vi "Parse Channels.vi"(4 "tx channel handle array":u32[](array[numeric]), 5 "ScheduledSDI":bool, 6 "rx channel handle array":u32[](array[numeric]), 7 "FIFO Idx Qs":T1, 8 "error in (no error)":errorcluster, 9 "Access":T3, 10 "Section GUID":string, 11 "Device Reference in":T2 format="%.0x") -> (0 "error out":errorcluster, 1 "Section BaseRate":i32, 2 "Section Data":T4[](array[typedef]) {"Labels Settings"."Label" format="%.0o"}, 3 "Device Reference out":T2 format="%.0x")   [LabVIEW 2011, in "AIT 429 Custom Device.lvlib"]
uses:
  AIT 429 Custom Device.lvlib
  RT Controls/RT HW Channel.ctl
  RT Controls/RT Label Settings.ctl
  Controls and Global/Label.ctl
  Controls and Global/transferPeriod.ctl
  RT Controls/Driver Data.ctl
  RT Controls/RT Word Settings.ctl
  <vilib>/NI Veristand/Custom Device API/Block Data Reference.ctl
  <vilib>/NI Veristand/Custom Device API/Data Reference.ctl
  RT Controls/RT Param Setting.ctl
  Controls and Global/Start Bit.ctl
  Controls and Global/Number of Bits.ctl
  Controls and Global/TransferType.ctl
  <vilib>/NI Veristand/Custom Device API/Data Access Type.ctl
  <vilib>/NI Veristand/Custom Device API/Custom Device Item Ref.ctl
  RT Controls/FIFO Idx Qs.ctl
  <vilib>/NI Veristand/Custom Device Tools/Custom Device Utility Library/NI VeriStand - Search for Item by GUID.vi
  Controls and Global/Global.vi
  <vilib>/NI Veristand/Custom Device API/Get Item Property (U16).vi
  <vilib>/NI Veristand/Custom Device API/Get Item Property (U32).vi
  <instrlib>/AIT 429/Public/Tx/Data/AIT 429 Set Scheduled Label Transfer Period.vi
  <vilib>/NI Veristand/Custom Device API/Get Item Property (Double).vi
  <vilib>/NI Veristand/Custom Device Tools/Custom Device Utility Library/Custom Device Utility Library.lvlib
  <vilib>/NI Veristand/Custom Device API/Custom Device API.lvlib
  <userlib>/ARINC-429/Owl429.lvlib
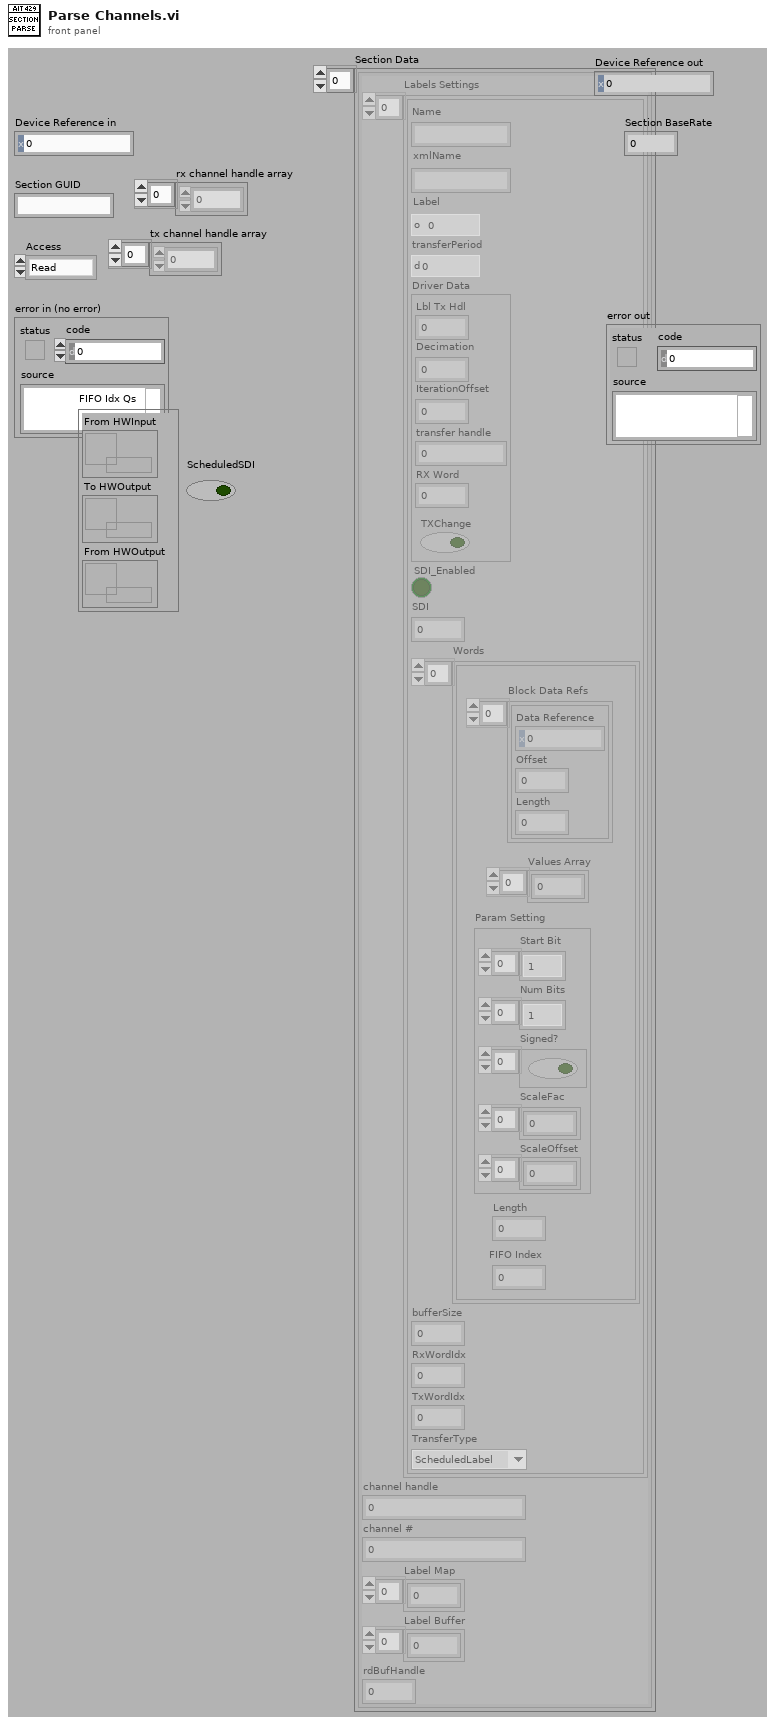
[diagram p1: front panel]
types:
  T1 = typedef "AIT 429 Custom Device.lvlib/FIFO Idx Qs.ctl" = cluster{"From HWInput":refnum<queue>, "To HWOutput":refnum<queue>, "From HWOutput":refnum<queue>}
  T2 = typedef "Custom Device API.lvlib/Custom Device Item Ref.ctl" = u64
  T3 = typedef "Custom Device API.lvlib/Data Access Type.ctl" = enum16{"Read", "Write"}
  T4 = typedef "AIT 429 Custom Device.lvlib/RT HW Channel.ctl" = cluster{"Labels Settings":T5[], "channel handle":u32, "channel #":u16, "Label Map":i32[], "Label Buffer":u32[], "rdBufHandle":u32}
  T5 = typedef "AIT 429 Custom Device.lvlib/RT Label Settings.ctl" = cluster{"Name":string, "xmlName":string, "Label":T6, "transferPeriod":T7, "Driver Data":T8, "SDI_Enabled":bool, "SDI":u8, "Words":T9[], "bufferSize":u32, "RxWordIdx":i32, "TxWordIdx":i32, "TransferType":T15}
  T6 = typedef "AIT 429 Custom Device.lvlib/Label.ctl" = u8
  T7 = typedef "AIT 429 Custom Device.lvlib/transferPeriod.ctl" = u32
  T8 = typedef "AIT 429 Custom Device.lvlib/Driver Data.ctl" = cluster{"Lbl Tx Hdl":u32, "Decimation":i32, "IterationOffset":i32, "transfer handle":u32, "RX Word":u32, "TXChange":bool}
  T9 = typedef "AIT 429 Custom Device.lvlib/RT Word Settings.ctl" = cluster{"Block Data Refs":T10[], "Values Array":dbl[], "Length":i32, "FIFO Index":i32, "Param Setting":T12}
  T10 = typedef "Custom Device API.lvlib/Block Data Reference.ctl" = cluster{"Data Reference":T11, "Offset":i32, "Length":i32}
  T11 = typedef "Custom Device API.lvlib/Data Reference.ctl" = i32
  T12 = typedef "AIT 429 Custom Device.lvlib/Rt Param Setting.ctl" = cluster{"Start Bit":T13[], "Num Bits":T14[], "Signed?":bool[], "ScaleFac":dbl[], "ScaleOffset":dbl[]}
  T13 = typedef "AIT 429 Custom Device.lvlib/Start Bit.ctl" = i32
  T14 = typedef "AIT 429 Custom Device.lvlib/Number of Bits.ctl" = i32
  T15 = typedef "AIT 429 Custom Device.lvlib/TransferType.ctl" = enum16{"ScheduledLabel", "Acyclic", "Block", "Strobe"}
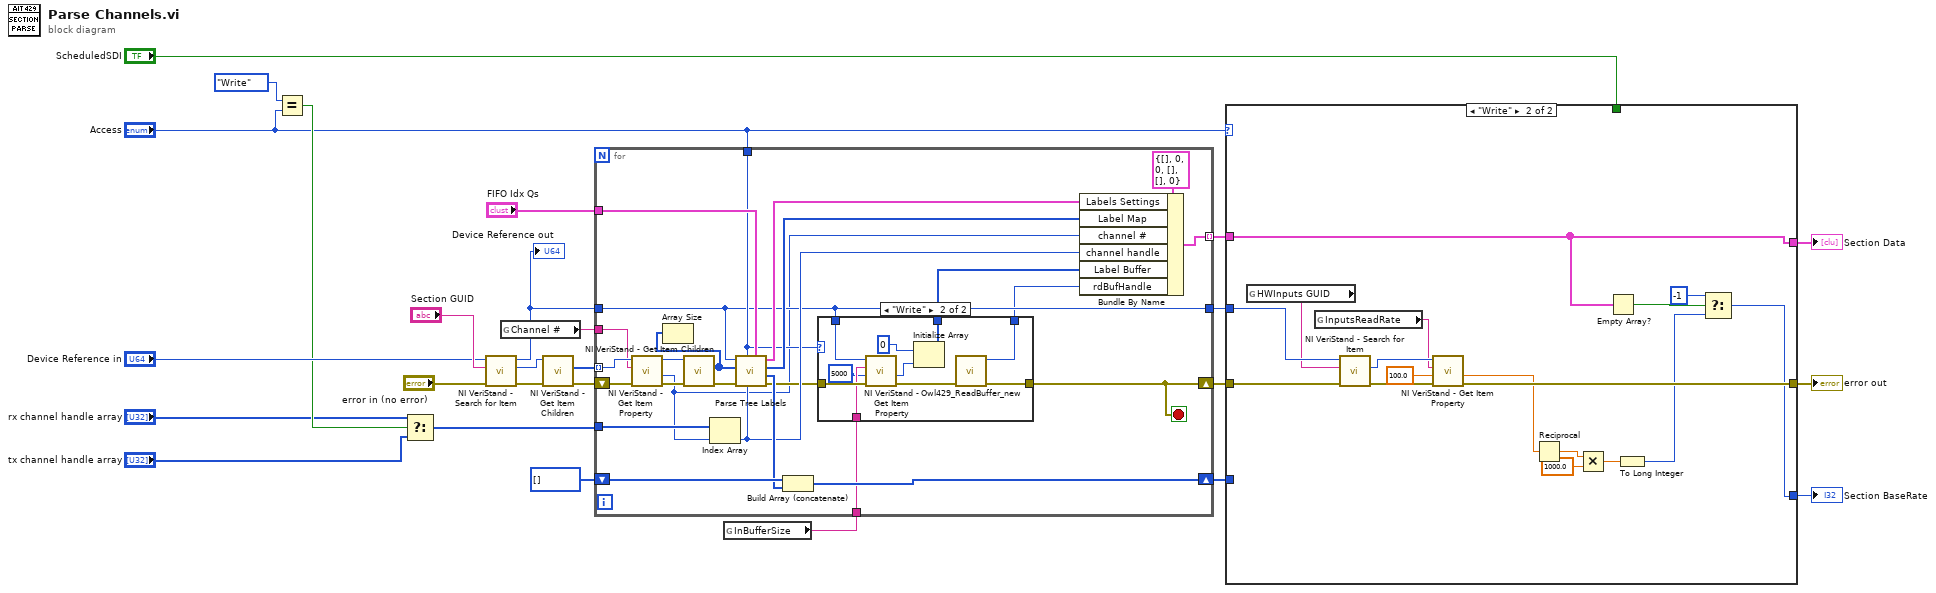
[diagram p0: block diagram]
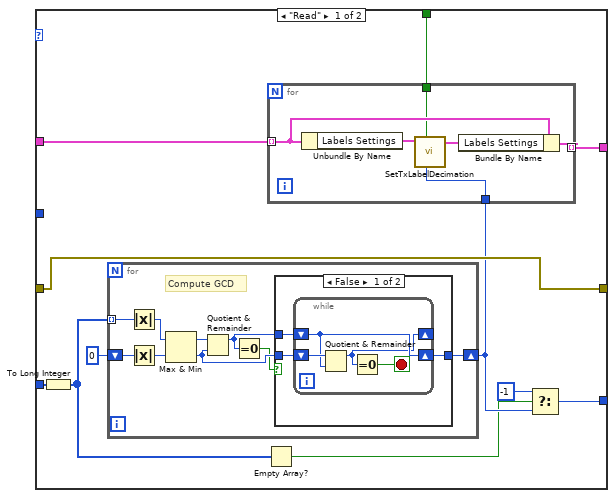
[diagram p2: hidden frame]
diagram:
  n1 = Equal?(x=Data_Access_Type."Write" ("y"), y="Access") -> (x = y?=w11:bool)
  n2 = Select(t="rx channel handle array", s=w11, f="tx channel handle array") -> (s? t:f=w8:u32[])
  n3 = call-poly <vilib>:"NI VeriStand - Search for Item.vi"("error in"="error in (no error)", "Item GUID"="Section GUID", "Section Ref in"="Device Reference in") -> ("error out"=w21:errorcluster, "Item Ref"=w22:T2, "Section Ref out"=w26:T2)  [unwired: 5 in, 1 out]
  "Device Reference out" <- w26
  n4 = global read "Global.vi" "Channel #"() -> (w3:string)
  n5 = call <vilib>:"NI VeriStand - Get Item Children.vi"("error in (no error)"=w21, "Item Ref in"=w22) -> ("error out"=w25:errorcluster, "Child Refs"=w24:T2[])  [unwired: 6 in, 2 out]
  n6 = global read "Global.vi" "InBufferSize"() -> (w2:string)
  n7 = for {
    tunnel: w24 -> [w42] mode=indexing
    tunnel: "Access" -> [w36]
    tunnel: w26 -> [w34]
    tunnel: [w49] -> w16 mode=indexing
    shift-right: [w30] -> w6
    shift-left: w25 -> [w44]
    shift-right: [w45] -> w17
    shift-left: u32[] [] -> [w47]
    tunnel: w8 -> [w39]
    tunnel: "FIFO Idx Qs" -> [w40]
    tunnel: [w34] -> w4
    tunnel: w3 -> [w33]
    tunnel: w2 -> [w32]
    stop <- w30 stop-if-true
    n8 = call-poly <vilib>:"NI VeriStand - Get Item Property.vi"("error in (no error)"=w44, "Property Name"=w33, "Item Ref in"=w42) -> ("error out"=w43:errorcluster, "Value"=w28:u16, "Item Ref out"=w41:T2)  [unwired: 5 in, 1 out]
    n9 = call <vilib>:"NI VeriStand - Get Item Children.vi"("error in (no error)"=w43, "Item Ref in"=w41) -> ("error out"=w48:errorcluster, "Child Refs"=w27:T2[])  [unwired: 6 in, 2 out]
    n10 = Array Size(array=w27) -> ()  [unwired: 1 out]
    n11 = Index Array(array=w39, index=w28) -> (element=w38:u32)
    n12 = call "Parse Tree Labels.vi"("FIFO Idx Qs"=w40, "Channel handle in"=w38, "Access"=w36, "error out"=w48, "Label Refs"=w27, "Custom Device Ref"=w34) -> ("error out"=w35:errorcluster, "Transfer Periods"=w46:u32[], "Label Map"=w37:i32[], "Label data"=w50:T5[])  [unwired: 2 in]
    n13 = Build Array (concatenate)(w47, w46) -> (w45:u32[])
    n14 = case shown="\"Write\"" w36 {
      tunnel: w35 -> [w52 w61]
      tunnel: w34 -> [_ w62]
      tunnel: w32 -> [_ w60]
      tunnel: [w52 w54] -> w30
      tunnel: [_ w56] -> w31
      tunnel: [_ w53] -> w29
      frame "Read", Default {
      }
      frame "Write" {
        n15 = call-poly <vilib>:"NI VeriStand - Get Item Property.vi"("error in (no error)"=w61, "Default Value"=u32 5000, "Property Name"=w60, "Item Ref in"=w62) -> ("error out"=w55:errorcluster, "Value"=w58:u32)  [unwired: 4 in, 2 out]
        n16 = Initialize Array(u32 0 ("element"), w58) -> (w56:u32[])
        n17 = call <userlib>:"Owl429_ReadBuffer_new.vi"("error in (no error)"=w55) -> ("error out"=w54:errorcluster, "buffer handle"=w53:u32)  [unwired: 9 in]
      }
    }
    n18 = Bundle By Name(cluster=T4 {"Labels Settings"=[], "channel handle"=0, "channel #"=0, "Label Map"=[], "Label Buffer"=[], "rdBufHandle"=0} ("HW Channel"), "Labels Settings"=w50, "Label Map"=w37, "channel #"=w28, "channel handle"=w38, "Label Buffer"=w31, "rdBufHandle"=w29) -> (w49:T4)
  }
  n19 = case shown="\"Write\"" "Access" {
    tunnel: w17 -> [w73 _]
    tunnel: w16 -> [w71 w100]
    tunnel: [w67 w97] -> w15
    tunnel: [w70 w100] -> w14
    tunnel: [w69 w107] -> w7
    tunnel: w6 -> [w69 w113]
    tunnel: w4 -> [_ w112]
    tunnel: "ScheduledSDI" -> [w68 _]
    frame "Read" {
      n20 = To Long Integer(number=w73) -> (32bit integer=w66:i32[])
      n21 = for {
        tunnel: w66 -> [w74] mode=indexing
        shift-right: [w76] -> w65
        shift-left: 0 ("gcd(x,y)") -> [w75]
        # "Compute GCD"
        n22 = Absolute Value(x=w74) -> (abs(x)=w81:i32)
        n23 = Absolute Value(x=w75) -> (abs(x)=w82:i32)
        n24 = Max & Min(x=w81, y=w82) -> (max(x,y)=w77:i32, min(x,y)=w79:i32)
        n25 = Quotient & Remainder(x=w77, y=w79) -> (x-y*floor(x/y)=w80:i32)  [unwired: 1 out]
        n26 = Equal To 0?(x=w80) -> (x = 0?=w78:bool)
        n27 = case shown="False" w78 {
          tunnel: [w85 w90] -> w76
          tunnel: w79 -> [w84 w90]
          tunnel: w80 -> [w83 _]
          frame False {
            n28 = while {
              shift-right: [w87] -> w85
              shift-left: w84 -> [w88]
              shift-right: [w86] -> _
              shift-left: w83 -> [w87]
              stop <- w89 stop-if-true
              n29 = Quotient & Remainder(x=w88, y=w87) -> (x-y*floor(x/y)=w86:i32)  [unwired: 1 out]
              n30 = Equal To 0?(x=w86) -> (x = 0?=w89:bool)
            }
          }
          frame True {
          }
        }
      }
      n31 = Empty Array?(array=w66) -> (empty?=w64:bool)
      n32 = for {
        tunnel: w71 -> [w95] mode=indexing
        tunnel: w65 -> [w92]
        tunnel: [w93] -> w70 mode=indexing
        tunnel: w68 -> [w91]
        n33 = Unbundle By Name(w95) -> ("Labels Settings"=w96:T5[])
        n34 = call "SetTxLabelDecimation.vi"("SectionBaseRate"=w92, "ScheduledSDI"=w91, "Labels Settings In"=w96) -> ("Label Settings Out"=w94:T5[])  [unwired: 7 in, 1 out]
        n35 = Bundle By Name(cluster=w95, "Labels Settings"=w94) -> (w93:T4)
      }
      n36 = Select(t=-1, s=w64, f=w65) -> (s? t:f=w67:i32)
    }
    frame "Write" {
      n37 = global read "Global.vi" "HWInputs GUID"() -> (w111:string)
      n38 = global read "Global.vi" "InputsReadRate"() -> (w108:string)
      n39 = call-poly <vilib>:"NI VeriStand - Search for Item.vi"("error in"=w113, "Item GUID"=w111, "Section Ref in"=w112) -> ("error out"=w110:errorcluster, "Item Ref"=w109:T2)  [unwired: 5 in, 2 out]
      n40 = call-poly <vilib>:"NI VeriStand - Get Item Property.vi"("error in (no error)"=w110, "Default Value"=100.0, "Property Name"=w108, "Item Ref in"=w109) -> ("error out"=w107:errorcluster, "Value"=w106:dbl)  [unwired: 4 in, 2 out]
      n41 = Reciprocal(x=w106) -> (1/x=w104:dbl)
      n42 = Multiply(x=w104, y=1000.0) -> (x*y=w102:dbl)
      n43 = Empty Array?(array=w100) -> (empty?=w99:bool)
      n44 = To Long Integer(number=w102) -> (32bit integer=w98:i32)
      n45 = Select(t=-1, s=w99, f=w98) -> (s? t:f=w97:i32)
    }
  }
  "Section Data" <- w14
  "error out" <- w7
  "Section BaseRate" <- w15
